vi "overlay_circular_fitting(SubVI).vi"(7 "Color":u32(colorbox)=16711680, 8 "error in (no error)":errorcluster, 9 "circle in":T1 {"Radius" format="%.2f"; "Center"."Y" format="%.2f"; "Center"."X" format="%.2f"}, 10 "points (pixel)":cluster{"X":sgl, "Y":sgl}[](array[cluster]), 11 "image dest":T2) -> (0 "error out":errorcluster, 2 "Circle out":T1 {"Radius" format="%.2f"; "Center"."Y" format="%.2f"; "Center"."X" format="%.2f"}, 3 "Image Out":T2)   [LabVIEW 2020]
uses:
  <vilib>/vision/Image Controls.llb/IMAQ Image.ctl
  <vilib>/vision/NI_Vision_Development_Module.lvlib
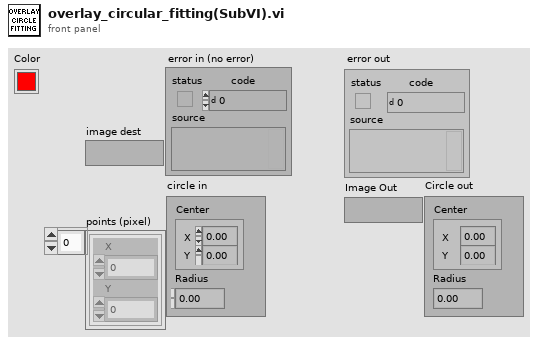
[diagram p1: front panel]
types:
  T1 = cluster{"Center":cluster{"X":sgl, "Y":sgl}, "Radius":dbl}
  T2 = typedef "IMAQ Image.ctl" = refnum<image>
  T3 = cluster{"Left":i32, "Top":i32, "Right":i32, "Bottom":i32}
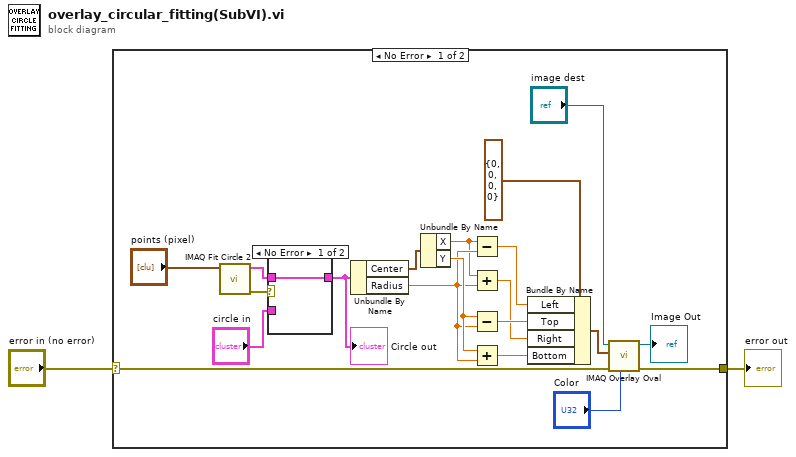
[diagram p0: block diagram]
diagram:
  n1 = case shown="No Error" "error in (no error)" {
    selector: "error in (no error)" -> [w8 w25]
    tunnel: [w10 w25] -> w2
    frame No Error {
      n2 = call "IMAQ Fit Circle 2"("Radial Points"="points (pixel)") -> ("error out"=w7:errorcluster, "Circle"=w6:T1)  [unwired: 5 in, 4 out]
      n3 = case shown="No Error" w7 {
        tunnel: w6 -> [w23 _]
        tunnel: [w23 w24] -> w5
        tunnel: "circle in" -> [_ w24]
        frame No Error {
        }
        frame Error {
        }
      }
      "Circle out" <- w5
      n4 = Unbundle By Name(w5) -> ("Center"=w12:cluster{"X":sgl, "Y":sgl}, "Radius"=w16:dbl)
      n5 = Unbundle By Name(w12) -> ("X"=w14:sgl, "Y"=w17:sgl)
      n6 = Subtract(x=w14, y=w16) -> (x-y=w15:dbl)
      n7 = Add(x=w14, y=w16) -> (x+y=w13:dbl)
      n8 = Subtract(x=w17, y=w16) -> (x-y=w18:dbl)
      n9 = Add(x=w17, y=w16) -> (x+y=w19:dbl)
      n10 = Bundle By Name(cluster=T3 {"Left"=0, "Top"=0, "Right"=0, "Bottom"=0} ("Bounding Rectangle"), "Left"=w15, "Top"=w18, "Right"=w13, "Bottom"=w19) -> (w21:T3)
      n11 = call "IMAQ Overlay Oval"("Color"="Color", "error in (no error)"=w8, "Bounding Rectangle"=w21, "Image"="image dest") -> ("error out"=w10:errorcluster, "Image Out"=→"Image Out":T2)  [unwired: 6 in]
    }
    frame Error {
    }
  }
  "error out" <- w2
